vi "ESP301_initandgetparams.vi"(0 "VISA resource name":refnum<visa-resource-name>, 1 "Error In":errorcluster) -> (2 "VISA resource name out":refnum<visa-resource-name>, 3 "Cluster":T1, 4 "Error Out":errorcluster)   [LabVIEW 2019]
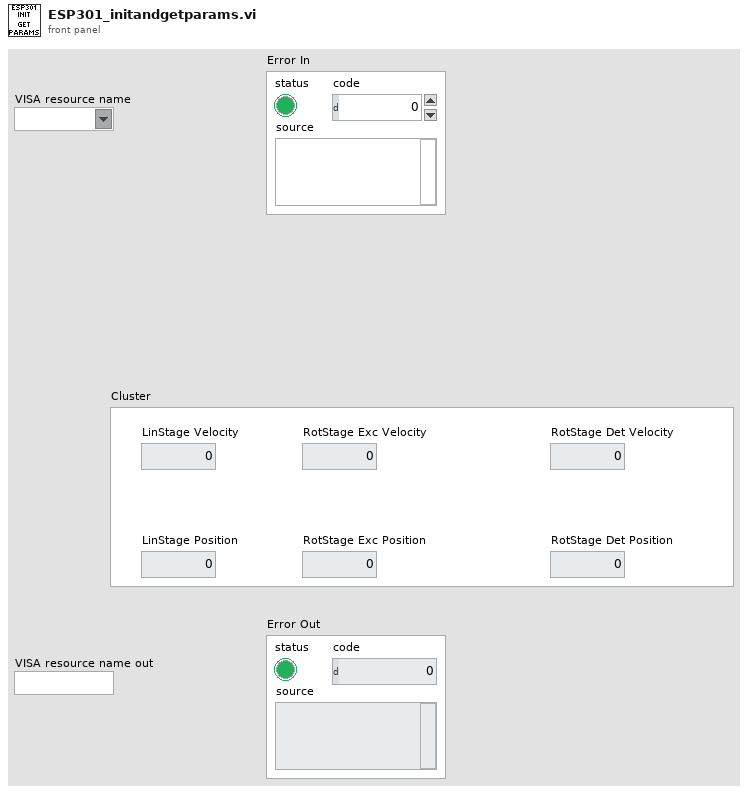
[diagram p1: front panel]
types:
  T1 = cluster{"LinStage Velocity":dbl, "RotStage Exc Velocity":dbl, "RotStage Det Velocity":dbl, "LinStage Position":dbl, "RotStage Exc Position":dbl, "RotStage Det Position":dbl}
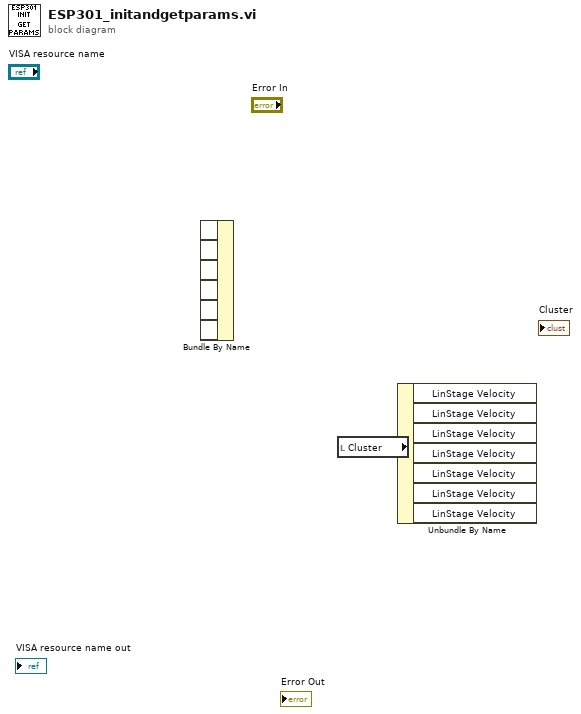
[diagram p0: block diagram]
diagram:
  n1 = Bundle By Name() -> ()  [unwired: 7 in, 1 out]
  n2 = local read "Cluster"() -> (w1:T1)
  n3 = Unbundle By Name(w1) -> ()  [unwired: 7 out]
